vi "Example Test 2.vi"(5 "b 2":dbl=4.0, 7 "a 2":dbl=3.0, 8 "error in (no error)":errorcluster, 10 "b":dbl=2.0, 11 "a":dbl=1.0) -> (0 "error out":errorcluster, 1 "myString":string, 2 "signal out 2":waveform(dbl), 3 "signal out":waveform(dbl), 6 "error out 2":errorcluster)   [LabVIEW 2014]
uses:
  <vilib>/measure/NI_MABase.lvlib
panel:
  in  "String control 1":string
  out "x+y":i32
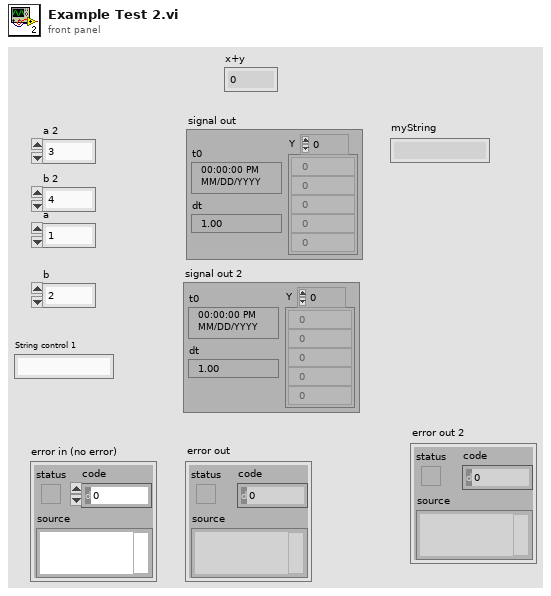
[diagram p1: front panel]
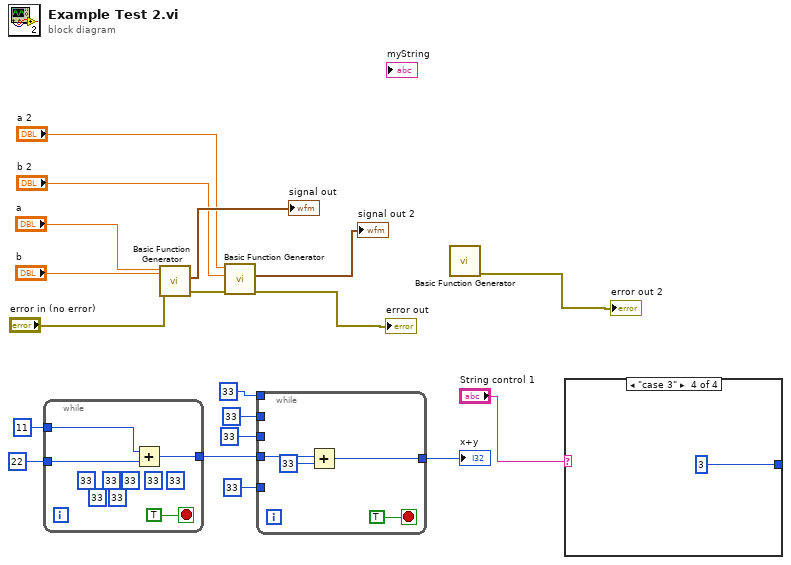
[diagram p0: block diagram]
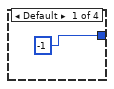
[diagram p2: hidden frame]
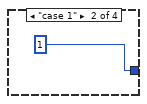
[diagram p3: hidden frame]
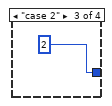
[diagram p4: hidden frame]
diagram:
  n1 = while {
    tunnel: 11 -> [w22]
    tunnel: 22 -> [w21]
    tunnel: [w20] -> w8
    stop <- TRUE stop-if-true
    (unwired) 33 ("y")
    (unwired) 33 ("y")
    (unwired) 33 ("y")
    (unwired) 33 ("y")
    (unwired) 33 ("y")
    (unwired) 33 ("y")
    (unwired) 33 ("y")
    n2 = Add(x=w22, y=w21) -> (x+y=w20:i32)
  }
  n3 = call <vilib>:"Basic Function Generator.vi"("error in (no error)"="error in (no error)", "amplitude"="b", "frequency"="a") -> ("error out"=w15:errorcluster, "signal out"=→"signal out":waveform(dbl))  [unwired: 6 in, 1 out]
  n4 = call <vilib>:"Basic Function Generator.vi"("error in (no error)"=w15, "amplitude"="b 2", "frequency"="a 2") -> ("error out"=→"error out":errorcluster, "signal out"=→"signal out 2":waveform(dbl))  [unwired: 6 in, 1 out]
  n5 = while {
    tunnel: w8 -> [w26]
    tunnel: [w24] -> w7
    tunnel: 33 ("y") -> [_]
    tunnel: 33 ("y") -> [_]
    tunnel: 33 ("y") -> [_]
    tunnel: 33 ("y") -> [_]
    stop <- TRUE stop-if-true
    n6 = Add(x=w26, y=33) -> (x+y=w24:i32)
  }
  "x+y" <- w7
  n7 = call <vilib>:"Basic Function Generator.vi"() -> ("error out"=→"error out 2":errorcluster)  [unwired: 9 in, 2 out]
  n8 = case shown="\"case 3\"" "String control 1" {
    tunnel: [-1 1 2 3] -> _
    frame Default {
    }
    frame "case 1" {
    }
    frame "case 2" {
    }
    frame "case 3" {
    }
  }
